vi "JSON Topology to Switch Driver Topology.vi"(8 "error in (no error)":errorcluster, 11 "Topology":T4) -> (0 "error out":errorcluster, 3 "Topologies":T1)   [LabVIEW 2015, in "SLSC Switch.lvlib" / "SLSC Switch.lvclass"]
uses:
  SLSC Switch.lvclass
  Controls/JSON.Topology.ctl
  Controls/JSON.InitialState.ctl
  Controls/JSON.ChannelList.ctl
  Controls/JSON.ConnectionList.ctl
  Controls/Topology.ctl
  Controls/MuxList Entry.ctl
  <vilib>/Utility/config.llb/NI_LVConfig.lvlib
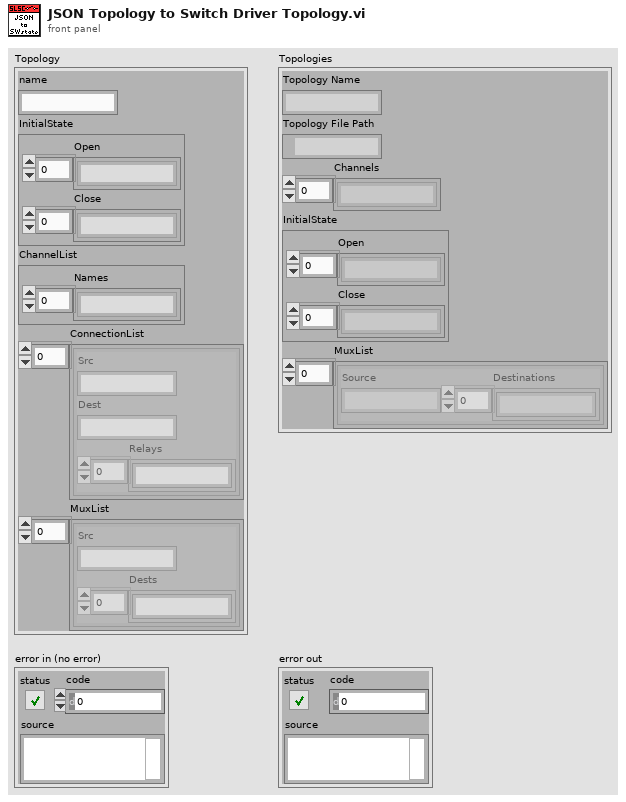
[diagram p1: front panel]
types:
  T1 = typedef "SLSC Switch.lvlib/SLSC Switch.lvclass/Topology.ctl" = cluster{"Topology Name":string, "Topology File Path":path, "Channels":string[], "InitialState":T2, "MuxList":T3[]}
  T2 = typedef "SLSC Switch.lvlib/SLSC Switch.lvclass/JSON.InitialState.ctl" = cluster{"Open":string[], "Close":string[]}
  T3 = typedef "SLSC Switch.lvlib/SLSC Switch.lvclass/MuxList Entry.ctl" = cluster{"Source":string, "Destinations":string[]}
  T4 = typedef "SLSC Switch.lvlib/SLSC Switch.lvclass/JSON.Topology.ctl" = cluster{"name":string, "InitialState":T2, "ChannelList":T5, "ConnectionList":T6[], "MuxList":cluster{"Src":string, "Dests":string[]}[]}
  T5 = typedef "SLSC Switch.lvlib/SLSC Switch.lvclass/JSON.ChannelList.ctl" = cluster{"Names":string[]}
  T6 = typedef "SLSC Switch.lvlib/SLSC Switch.lvclass/JSON.ConnectionList.ctl" = cluster{"Src":string, "Dest":string, "Relays":string[]}
  T7 = typedef "NI_LVConfig.lvlib/Config Data RefNum.ctl" = refnum<k1>
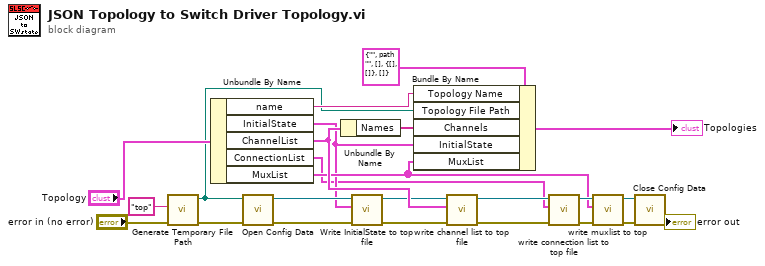
[diagram p0: block diagram]
diagram:
  n1 = call <vilib>:"Generate Temporary File Path.vi"("error in (no error)"="error in (no error)", "Temporary File Extension (tmp)"="top") -> ("error out"=w3:errorcluster, "Unique Temporary File Path"=w4:path)  [unwired: 8 in]
  n2 = Unbundle By Name("Topology") -> ("name"=w11:string, "InitialState"=w12:T2, "ChannelList"=w24:T5, "ConnectionList"=w8:T6[], "MuxList"=w13:cluster{"Src":string, "Dests":string[]}[])
  n3 = call <vilib>:"Open Config Data.vi"("error in (no error)"=w3, "configuration file path"=w4) -> ("error out"=w10:errorcluster, "refnum"=w21:T7)  [unwired: 7 in, 1 out]
  n4 = Unbundle By Name(w24) -> ("Names"=w23:string[])
  n5 = call "Write InitialState to top file.vi"("error in (no error)"=w10, "InitialState"=w12, "Refnum in"=w21) -> ("error out"=w7:errorcluster, "Refnum out"=w15:T7)  [unwired: 7 in]
  n6 = Bundle By Name(cluster=T1 {"Topology Name"="", "Topology File Path"=path "", "Channels"=[], "InitialState"={"Open"=[], "Close"=[]}, "MuxList"=[]} ("Topologies"), "Topology Name"=w11, "Topology File Path"=w4, "Channels"=w23, "InitialState"=w12, "MuxList"=w13) -> (→"Topologies":T1)
  n7 = call "write channel list to top file.vi"("error in (no error)"=w7, "ChannelList"=w24, "Refnum in"=w15) -> ("error out"=w9:errorcluster, "Refnum out"=w16:T7)  [unwired: 7 in]
  n8 = call "write connection list to top file.vi"("error in (no error)"=w9, "ConnectionList"=w8, "Refnum in"=w16) -> ("error out"=w20:errorcluster, "Refnum out"=w19:T7)  [unwired: 7 in]
  n9 = call "write muxlist to top.vi"("error in (no error)"=w20, "MuxList"=w13, "Refnum in"=w19) -> ("error out"=w18:errorcluster, "Refnum out"=w17:T7)  [unwired: 7 in]
  n10 = call <vilib>:"Close Config Data.vi"("error in (no error)"=w18, "refnum"=w17) -> ("error out"=→"error out":errorcluster)  [unwired: 8 in, 1 out]
